vi "ExternalIO Port Names.vi"(8 "error in (no error)":errorcluster) -> (0 "error out":errorcluster, 3 "Ports Out":string[](array[string]))   [LabVIEW 2011]
uses:
  SesWrapper/SesWrapper.lvlib
panel:
  in  "Ports":string[](array[string])
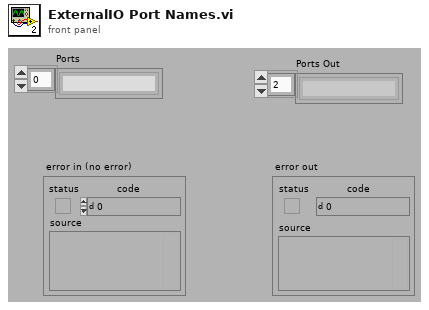
[diagram p1: front panel]
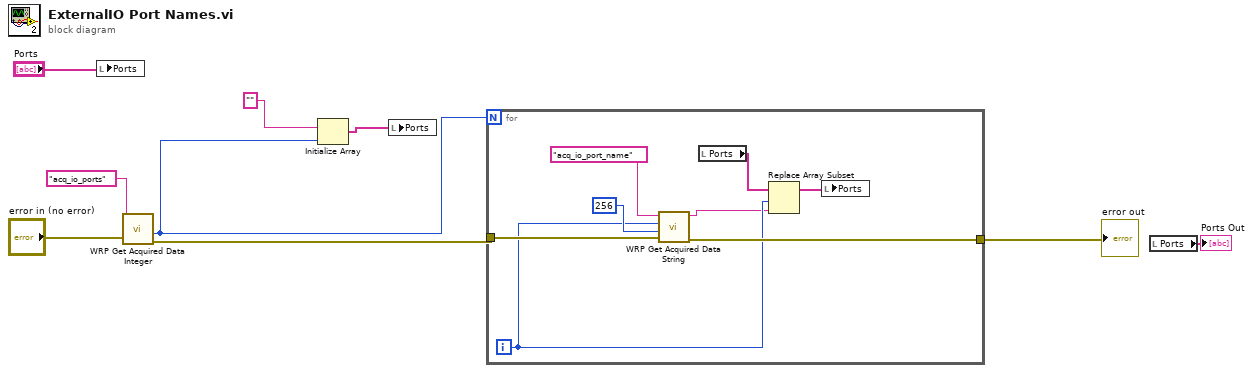
[diagram p0: block diagram]
diagram:
  n1 = local write "Ports"("Ports") -> ()
  n2 = call "WRP Get Acquired Data Integer.vi"("error in (no error)"="error in (no error)", "parameter"="acq_io_ports") -> ("error out"=w8:errorcluster, "size out"=w1:i32)  [unwired: 6 in, 2 out]
  n3 = Initialize Array("", w1) -> (w3:string[])
  n4 = local write "Ports"(w3) -> ()
  n5 = for {
    N: w1 -> [_]
    tunnel: w8 -> [w16]
    tunnel: [w15] -> w5
    i -> [w12]
    n6 = call "WRP Get Acquired Data String.vi"("error in (no error)"=w16, "size"=256, "index"=w12, "parameter"="acq_io_port_name") -> ("error out"=w15:errorcluster, "data"=w11:string)  [unwired: 4 in, 2 out]
    n7 = local read "Ports"() -> (w13:string[])
    n8 = Replace Array Subset(array=w13, new element=w11, index=w12) -> (w10:string[])
    n9 = local write "Ports"(w10) -> ()
  }
  "error out" <- w5
  n10 = local read "Ports"() -> (→"Ports Out":string[])
